vi "StrikerNormal.vi"(6 "atacando ao contrário?":bool=TRUE, 7 "AI Parameters":T1={"GotoKick"={"Dist do cone a frente"=150.0, "attacker farback"=1500.0, "Perto"=300.0, "min dist to kick"=150.0, "kick eps"=0.0, "Time to transition"=0.05}, "Attacker"={"CC chute"=0.09, "CC passe"=0.045, "Kick Force"=100.0, "D ball-robot Kick"=200.0, "D ball-robot Pass"=0.3}, "Defender"={"D max"=1700.0, "Vel p/ robô av"=1000.0, "Kick Force"=100.0, "D atk-def"=0.0, "D farback"=0.0}, "Timeout"={"Field/v in x"=6.0, "Dist Robots"=300, "Dist up in y"=300}, "Pose Striker"={"dist"=200.0, "Numeric"=-4.0, "dist 2"=200.0}, "Dist Stop"=300.0, "Distance when ball out"=200, "D central gap "=150.0} {"D central gap" format="%#_13g"; "Dist Stop" format="%#_13g"; "Pose Striker"."Numeric" format="%#_13g"; "Defender"."Kick Force" format="%#_13g"; "Defender"."Vel p/ robô av" format="%#_13g"; "Attacker"."D ball-robot Kick" format="%#_13g"; "Attacker"."Kick Force" format="%#_13g"; "Attacker"."CC passe" format="%#_13g"; "Attacker"."CC chute" format="%#_13g"; "GotoKick"."kick eps" format="%#_13g"; "GotoKick"."min dist to kick" format="%#_13g"; "GotoKick"."Perto" format="%#_13g"; "GotoKick"."attacker farback" format="%#_13g"; "GotoKick"."Dist do cone a frente" format="%#_13g"}, 8 "IA Input":T7={"our_robots"=[], "enemy_robots"=[], "balls"=[], "geometry"={"line_width"=0, "field_length"=0, "field_width"=0, "boundary_width"=0, "referee_width"=0, "goal_width"=0, "goal_depth"=0, "goal_wall_width"=0, "center_circle_radius"=0, "defense_radius"=0, "defense_stretch"=0, "free_kick_from_defense_dist"=0, "penalty_spot_from_field_line_dist"=0, "penalty_line_from_spot_dist"=0}, "IA Judge"={"stage"="", "command"="", "our_goalie_id"=0.0, "enemy_goalie_id"=0.0, "command enum"=enum."Halt", "Time"=enum."Azul"}, "Received Timestamp"=timestamp(0 s since 1904-01-01), "Events"={"Touch"=FALSE, "Ball out"=FALSE, "id touch"=0.0, "Ball out of \nVision"=FALSE, "Ball inside \nGoalie area"=FALSE, "Robot not responding"=FALSE, "Robots responding status"=[1.0, 1.0, 1.0, 1.0, 1.0, 1.0], "Enemy Ball \nPossession"=FALSE, "Pass State"=FALSE, "id end of pass"=0.0, "Kick"=FALSE, "Id Possession"=0.0}}, 9 "balls":T5[](array[typedef])=[{"x"=-2165.869384765625, "y"=510.4085693359375, "timestamp"=timestamp(2082758857.4639893 s since 1904-01-01), "Vel_x"=0.0, "Vel_y"=0.0, "Pos Bola Est"=[]}], 10 "Field Size in":T6={"line_width"=10, "field_length"=6000, "field_width"=4000, "boundary_width"=250, "referee_width"=425, "goal_width"=700, "goal_depth"=180, "goal_wall_width"=20, "center_circle_radius"=500, "defense_radius"=500, "defense_stretch"=350, "free_kick_from_defense_dist"=700, "penalty_spot_from_field_line_dist"=450, "penalty_line_from_spot_dist"=350}, 11 "Robot in":T2={"id"=5, "function"=enum."Attacker", "x"=-1842.5054931640625, "y"=520.60986328125, "orientation"=-2.7555055618286133, "v_tangent"=0.0, "v_normal"=0.0, "v_ang"=0.0, "kick_x"=0.0, "kick_z"=0.0, "dribble"=FALSE, "Timestamp"=timestamp(2082758857.4639893 s since 1904-01-01), "dest_x"=0.0, "dest_y"=0.0, "dest_orientation"=0.0, "estimatives"={"est_v_tangent"=0.0, "est_v_normal"=0.0, "est_vx"=0.0, "est_vy"=0.0, "Pos Robot Est"=[]}, "dest_x_kick"=0.0, "dest_y_kick"=0.0, "Gap Coord"=[], "States"=enum."GoToTangent"}) -> (2 "Robot out":T2={"id"=5, "function"=enum."Attacker", "x"=-1842.5054931640625, "y"=520.60986328125, "orientation"=-2.7555055618286133, "v_tangent"=-0.08361641967936218, "v_normal"=-0.20513016702014014, "v_ang"=0.24456003022714357, "kick_x"=0.0, "kick_z"=0.0, "dribble"=FALSE, "Timestamp"=timestamp(2082758857.4639893 s since 1904-01-01), "dest_x"=0.0, "dest_y"=0.0, "dest_orientation"=0.0, "estimatives"={"est_v_tangent"=0.0, "est_v_normal"=0.0, "est_vx"=0.0, "est_vy"=0.0, "Pos Robot Est"=[]}, "dest_x_kick"=0.0, "dest_y_kick"=0.0, "Gap Coord"=[], "States"=enum."GoToTangent"})   [LabVIEW 2016]
uses:
  Core/AI Robot.ctl
  Functions Enum.ctl
  AttackerStates.ctl
  Core/AI Input.ctl
  Core/AI Ball.ctl
  Core/Field Size.ctl
  Core/AI Judge.ctl
  Command Enum.ctl
  Util/Events/Events.ctl
  AI Parameters.ctl
panel:
  in  "IDattacker":dbl
  in  "Yattacker":dbl
  in  "Xattacker":dbl
  out "States":T4
  out "sentido":dbl
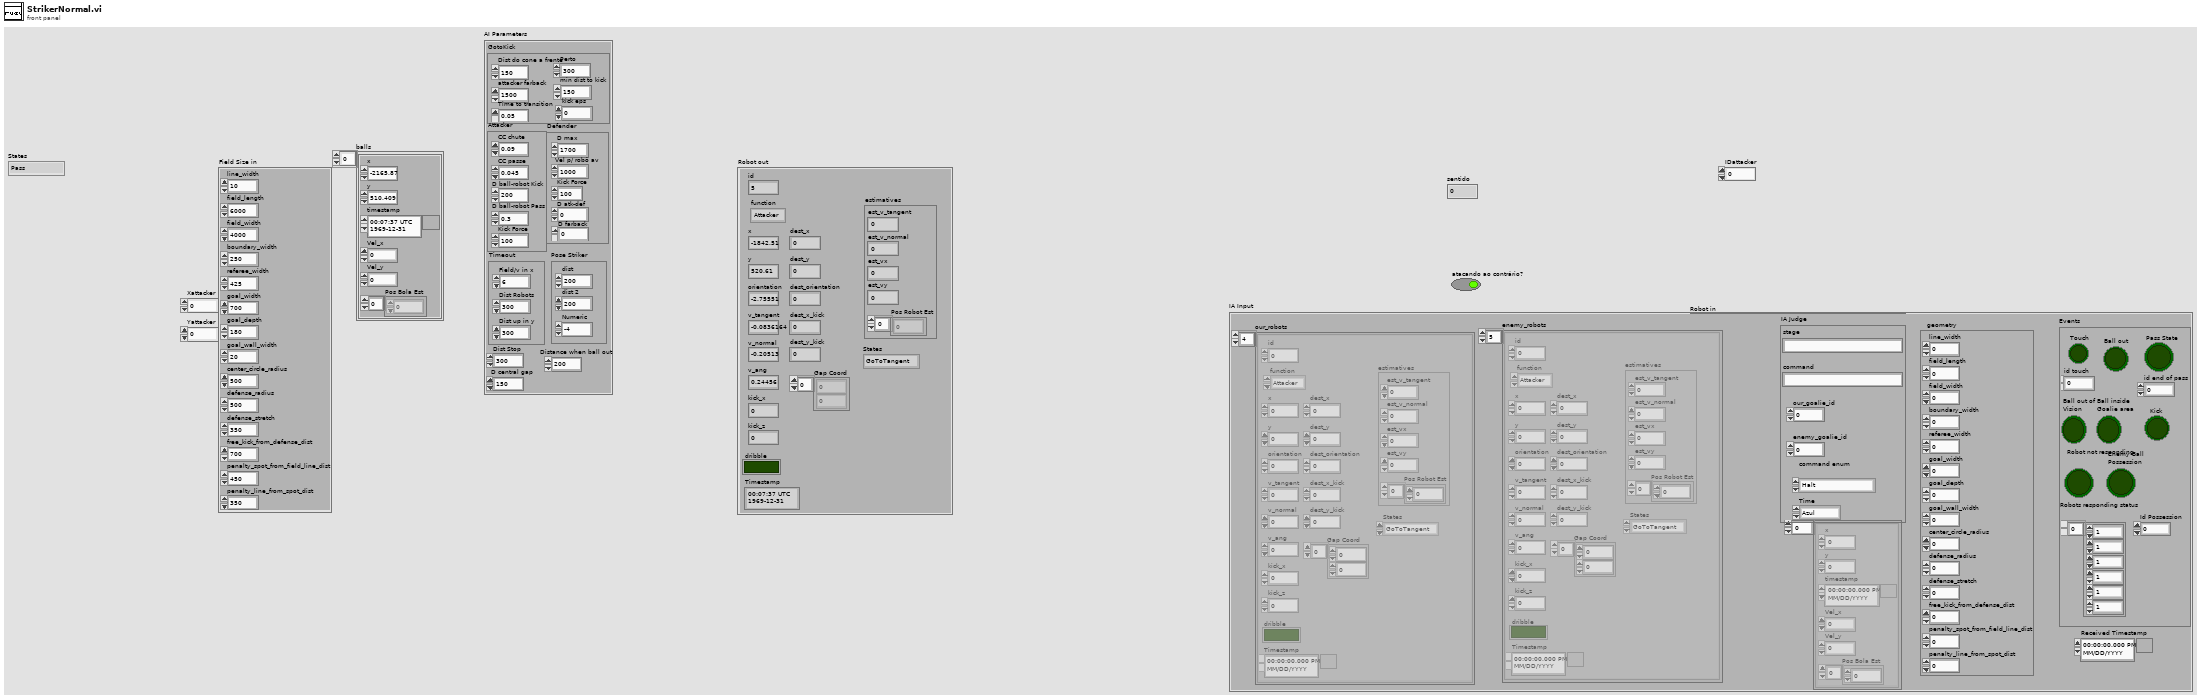
[diagram p1: front panel]
types:
  T1 = typedef "AI Parameters.ctl" = cluster{"GotoKick":cluster{"Dist do cone a frente":dbl, "attacker farback":dbl, "Perto":dbl, "min dist to kick":dbl, "kick eps":dbl, "Time to transition":dbl}, "Attacker":cluster{"CC chute":dbl, "CC passe":dbl, "Kick Force":dbl, "D ball-robot Kick":dbl, "D ball-robot Pass":dbl}, "Defender":cluster{"D max":dbl, "Vel p/ robô av":dbl, "Kick Force":dbl, "D atk-def":dbl, "D farback":dbl}, "Timeout":cluster{"Field/v in x":dbl, "Dist Robots":u32, "Dist up in y":u32}, "Pose Striker":cluster{"dist":dbl, "Numeric":dbl, "dist 2":dbl}, "Dist Stop":dbl, "Distance when ball out":i32, "D central gap ":dbl}
  T2 = typedef "AI Robot.ctl" = cluster{"id":u32, "function":T3, "x":dbl, "y":dbl, "orientation":dbl, "v_tangent":dbl, "v_normal":dbl, "v_ang":dbl, "kick_x":dbl, "kick_z":dbl, "dribble":bool, "Timestamp":timestamp, "dest_x":dbl, "dest_y":dbl, "dest_orientation":dbl, "estimatives":cluster{"est_v_tangent":dbl, "est_v_normal":dbl, "est_vx":dbl, "est_vy":dbl, "Pos Robot Est":dbl[]}, "dest_x_kick":dbl, "dest_y_kick":dbl, "Gap Coord":dbl[], "States":T4}
  T3 = typedef "Functions Enum.ctl" = enum16{"Attacker", "Goalie", "Defender", "Striker", "Goto 0", "Dummy", "Kicker", "ZigZag"}
  T4 = typedef "AttackerStates.ctl" = enum16{"Pass", "GoToTangent", "BallGetting", "GoToKick", ""}
  T5 = typedef "AI Ball.ctl" = cluster{"x":dbl, "y":dbl, "timestamp":timestamp, "Vel_x":dbl, "Vel_y":dbl, "Pos Bola Est":dbl[]}
  T6 = typedef "Field Size.ctl" = cluster{"line_width":u32, "field_length":u32, "field_width":u32, "boundary_width":u32, "referee_width":u32, "goal_width":u32, "goal_depth":u32, "goal_wall_width":u32, "center_circle_radius":u32, "defense_radius":u32, "defense_stretch":u32, "free_kick_from_defense_dist":u32, "penalty_spot_from_field_line_dist":u32, "penalty_line_from_spot_dist":u32}
  T7 = typedef "AI Input.ctl" = cluster{"our_robots":T2[], "enemy_robots":T2[], "balls":T5[], "geometry":T6, "IA Judge":T8, "Received Timestamp":timestamp, "Events":T10}
  T8 = typedef "AI Judge.ctl" = cluster{"stage":string, "command":string, "our_goalie_id":dbl, "enemy_goalie_id":dbl, "command enum":T9, "Time":enum16{"Azul", "Amarelo"}}
  T9 = typedef "Command Enum.ctl" = enum16{"Halt", "Stop", "Force Start", "PKA Normal Start", "Prepare Kickoff Ally", "PKE Normal Start", "Prepare Kickoff Enemy", "Prepare Penalty Ally", "PPA Normal Start", "Prepare Penalty Enemy", "PPE Normal Start", "Direct Free Enemy", "Direct Free Ally", "Indirect Free Enemy", "Indirect Free Ally", "Timeout Enemy", "Timeout Ally", "Goal Enemy", "Goal Ally", "Ball Placement Enemy", "Ball Placement Ally", "Normal Half Time", "Extra Time Break", "Extra Half Time", "None"}
  T10 = typedef "Events.ctl" = cluster{"Touch":bool, "Ball out":bool, "id touch":dbl, "Ball out of \nVision":bool, "Ball inside \nGoalie area":bool, "Robot not responding":bool, "Robots responding status":dbl[], "Enemy Ball \nPossession":bool, "Pass State":bool, "id end of pass":dbl, "Kick":bool, "Id Possession":dbl}
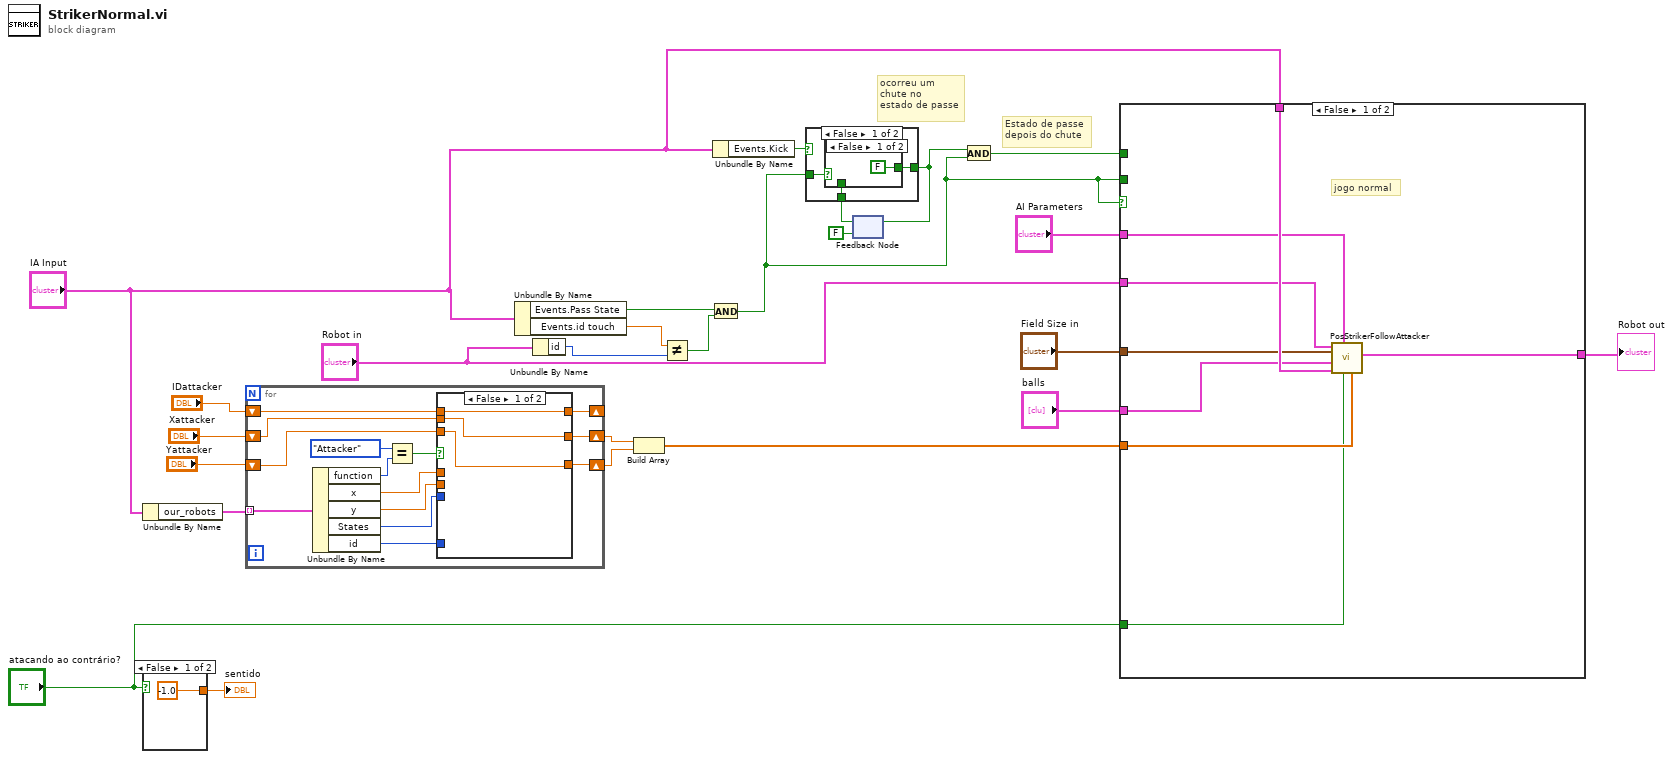
[diagram p0: block diagram]
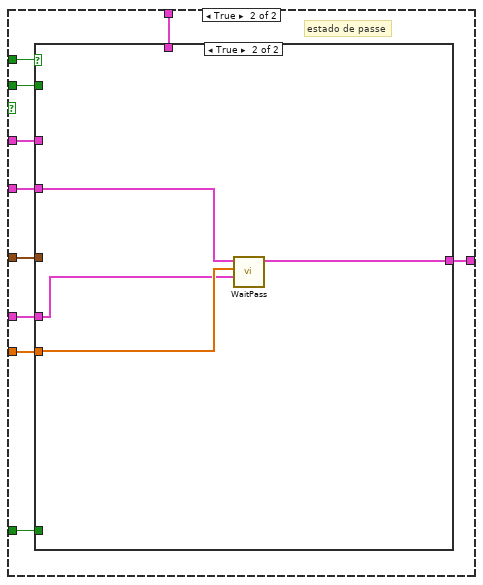
[diagram p2: hidden frame]
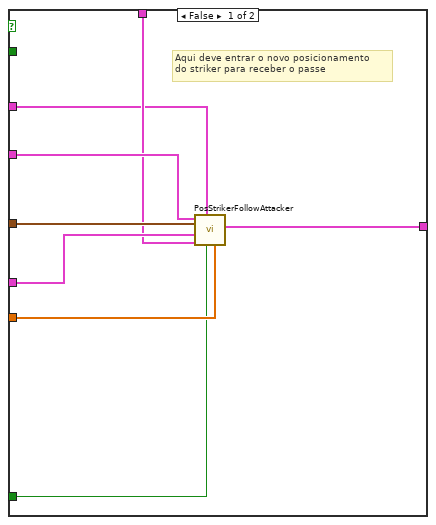
[diagram p3: hidden frame]
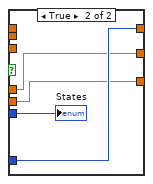
[diagram p4: hidden frame]
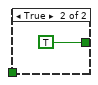
[diagram p6: hidden frame]
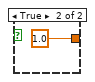
[diagram p7: hidden frame]
diagram:
  # "ocorreu um \nchute no\nestado de passe"
  # "Estado de passe\ndepois do chute"
  n1 = Unbundle By Name("IA Input") -> ("our_robots"=w18:T2[])
  n2 = case shown="False" "atacando ao contrário?" {
    tunnel: [-1.0 1.0] -> w25
    frame False {
    }
    frame True {
    }
  }
  "sentido" <- w25
  n3 = for {
    tunnel: w18 -> [w36] mode=indexing
    shift-right: [w32] -> w14
    shift-left: "Xattacker" -> [w30]
    shift-right: [w31] -> w13
    shift-left: "Yattacker" -> [w29]
    shift-right: [w33] -> _
    shift-left: "IDattacker" -> [w28]
    n4 = Unbundle By Name(w36) -> ("function"=w41:T3, "x"=w38:dbl, "y"=w37:dbl, "States"=w35:T4, "id"=w34:u32)
    n5 = Equal?(x=Functions_Enum."Attacker", y=w41) -> (x = y?=w39:bool)
    n6 = case shown="False" w39 {
      tunnel: w38 -> [_ w46]
      tunnel: w37 -> [_ w45]
      tunnel: w35 -> [_ w48]
      tunnel: w34 -> [_ w47]
      tunnel: [w42 w47] -> w33
      tunnel: [w44 w46] -> w32
      tunnel: [w43 w45] -> w31
      tunnel: w30 -> [w44 _]
      tunnel: w29 -> [w43 _]
      tunnel: w28 -> [w42 _]
      frame False {
      }
      frame True {
        "States" <- w48
      }
    }
  }
  n7 = Unbundle By Name("IA Input") -> ("Events.Pass State"=w19:bool, "Events.id touch"=w5:dbl)
  n8 = Unbundle By Name("Robot in") -> ("id"=w3:u32)
  n9 = Build Array(w14, w13) -> (w12:dbl[])
  n10 = Not Equal?(x=w5, y=w3) -> (x != y?=w6:bool)
  n11 = And(x=w19, y=w6) -> (x .and. y?=w7:bool)
  n12 = Unbundle By Name("IA Input") -> ("Events.Kick"=w24:bool)
  n13 = feedback #1(FALSE) -> (w22:bool)
  n14 = case shown="False" w24 {
    tunnel: [w50 TRUE] -> w23
    tunnel: w22 -> [w49 _]
    tunnel: w7 -> [w51 _]
    frame False {
      n15 = case shown="False" w51 {
        tunnel: [FALSE w53] -> w50
        tunnel: w49 -> [_ w53]
        frame False {
        }
        frame True {
        }
      }
    }
    frame True {
    }
  }
  n16 = feedback-in #1(w23) -> ()
  n17 = And(x=w23, y=w7) -> (x .and. y?=w20:bool)
  n18 = case shown="False" w7 {
    tunnel: w20 -> [_ w64]
    tunnel: w7 -> [_ w65]
    tunnel: "Robot in" -> [w61 w72]
    tunnel: w12 -> [w58 w71]
    tunnel: "atacando ao contrário?" -> [w57 w70]
    tunnel: "Field Size in" -> [w60 w69]
    tunnel: "balls" -> [w59 w68]
    tunnel: "IA Input" -> [w62 w67]
    tunnel: [w56 w66] -> w8
    tunnel: "AI Parameters" -> [w55 w63]
    frame False {
      # "jogo normal"
      n19 = call "PosStrikerFollowAttacker.vi"("Pos Attacker"=w58, "atacando ao contrário?"=w57, "AI Parameters"=w55, "IA Input"=w62, "balls"=w59, "Field Size in"=w60, "Robot in"=w61) -> ("Robot out"=w56:T2)  [unwired: 4 in]
    }
    frame True {
      # "estado de passe"
      n20 = case shown="True" w64 {
        tunnel: w65 -> [_ _]
        tunnel: w72 -> [w78 w84]
        tunnel: w71 -> [w80 w83]
        tunnel: [w74 w82] -> w66
        tunnel: w70 -> [w79 _]
        tunnel: w69 -> [w77 _]
        tunnel: w68 -> [w76 w81]
        tunnel: w67 -> [w75 _]
        tunnel: w63 -> [w73 _]
        frame False {
          # "Aqui deve entrar o novo posicionamento\ndo striker para receber o passe"
          n21 = call "PosStrikerFollowAttacker.vi"("Pos Attacker"=w80, "atacando ao contrário?"=w79, "AI Parameters"=w73, "IA Input"=w75, "balls"=w76, "Field Size in"=w77, "Robot in"=w78) -> ("Robot out"=w74:T2)  [unwired: 4 in]
        }
        frame True {
          n22 = call "WaitPass.vi"("balls"=w81, "Target"=w83, "Robot in"=w84) -> ("Robot out"=w82:T2)  [unwired: 8 in]
        }
      }
    }
  }
  "Robot out" <- w8
